vi "imagesurfacetest.vi"(10 "ROilevel":T1, 11 "ImageSrc":T2) -> (3 "ImageDst":T2(plugin-control))   [LabVIEW 2015]
uses:
  <vilib>/vision/Image Controls.llb/IMAQ Image.ctl
  ImageSurface.dll
  <vilib>/vision/NI_Vision_Development_Module.lvlib
panel:
  in  "Radius":i32=20
  in  "valueMin":i16
  in  "valueMax":i16=10000
  in  "SkipInvalidValue":bool=TRUE
  out "Return":i32
  out "Alpha 2":dbl=0.09707686755683868
  out "Beta 2":dbl=-0.07680741008059666
  out "Gamma 2":dbl=1309.996631781547
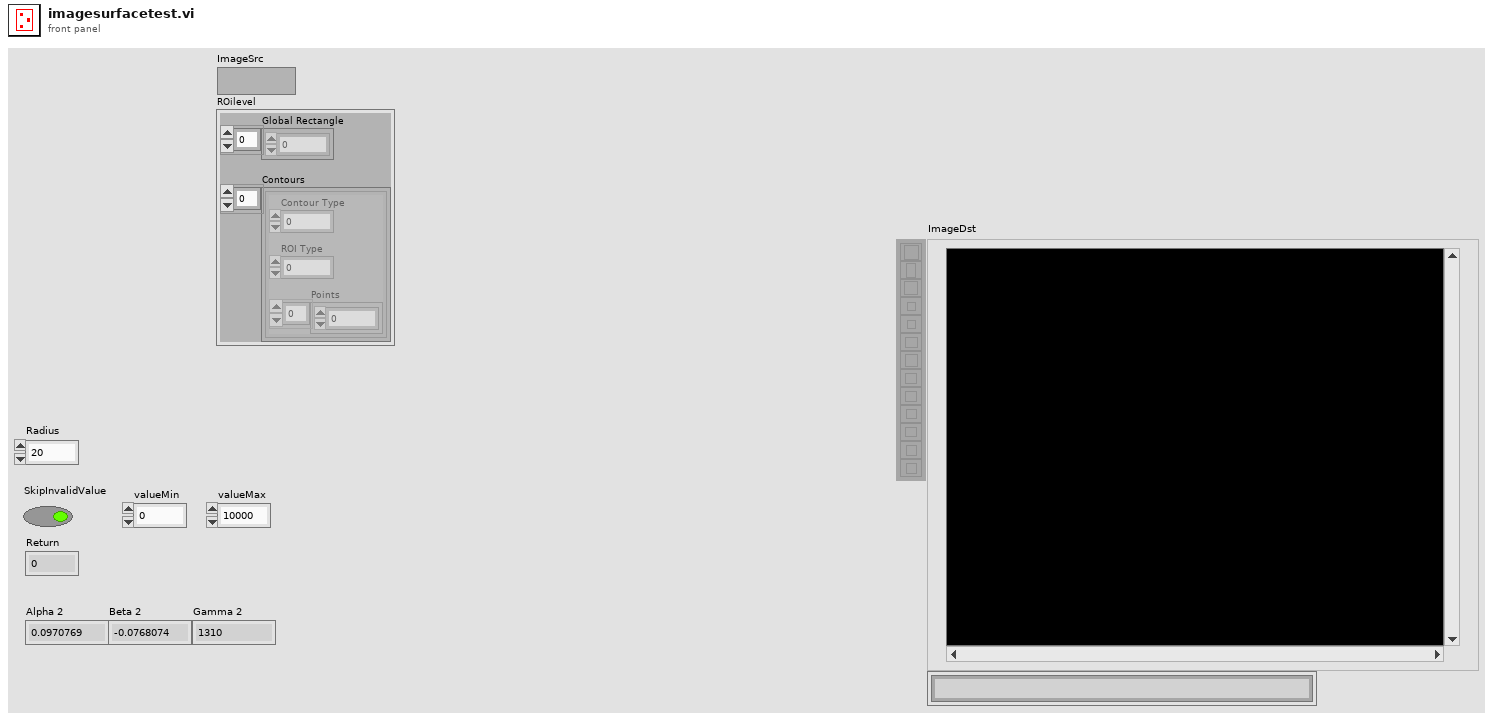
[diagram p1: front panel]
types:
  T1 = cluster{"Global Rectangle":i32[], "Contours":cluster{"Contour Type":u32, "ROI Type":u32, "Points":i32[]}[]}
  T2 = typedef "IMAQ Image.ctl" = refnum<image>
  T3 = cluster{"Contour Type":u32, "ROI Type":u32, "Points":i32[]}[]
  T4 = cluster{"Contour Type":u32, "ROI Type":u32, "Points":i32[]}
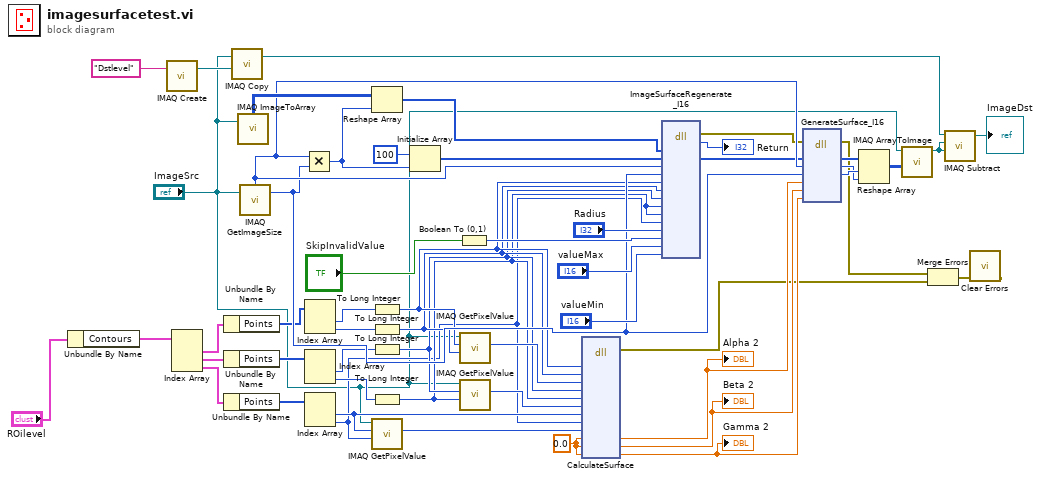
[diagram p0: block diagram]
diagram:
  w24 = 0.0 ("Gamma")
  n1 = Unbundle By Name("ROilevel") -> ("Contours"=w22:T3)
  n2 = call "IMAQ Create"("Image Name"="Dstlevel") -> ("New Image"=w7:T2)  [unwired: 4 in, 1 out]
  n3 = Index Array(array=w22) -> (element #1=w21:T4, element #2=w15:T4, element #3=w14:T4)  [unwired: 3 in]
  n4 = Unbundle By Name(w21) -> ("Points"=w20:i32[])
  n5 = Unbundle By Name(w15) -> ("Points"=w17:i32[])
  n6 = Unbundle By Name(w14) -> ("Points"=w16:i32[])
  n7 = call "IMAQ Copy"("Image Dst"=w7, "Image Src"="ImageSrc") -> ("Image Dst Out"=w5:T2)  [unwired: 4 in, 1 out]
  n8 = call "IMAQ ImageToArray"("Image"="ImageSrc") -> ("Image Pixels (U8)"=w53:u8[][])  [unwired: 3 in, 4 out]
  n9 = call "IMAQ GetImageSize"("Image"="ImageSrc") -> ("Y Resolution"=w35:i32, "X Resolution"=w36:i32)  [unwired: 3 in, 1 out]
  n10 = Multiply(x=w36, y=w35) -> (x*y=w45:i32)
  n11 = Index Array(array=w20) -> (element #1=w19:i32, element #2=w18:i32)  [unwired: 2 in]
  n12 = Index Array(array=w17) -> (element #1=w13:i32, element #2=w12:i32)  [unwired: 2 in]
  n13 = Index Array(array=w16) -> (element #1=w11:i32, element #2=w10:i32)  [unwired: 2 in]
  n14 = Reshape Array(w53, w45) -> (w48:u8[])
  n15 = To Long Integer(number=w19) -> (32bit integer=w28:i32)
  n16 = To Long Integer(number=w18) -> (32bit integer=w27:i32)
  n17 = To Long Integer(number=w13) -> (32bit integer=w26:i32)
  n18 = To Long Integer(number=w12) -> (32bit integer=w25:i32)
  n19 = call "IMAQ GetPixelValue"("Image"="ImageSrc", "X Coordinate"=w11, "Y Coordinate"=w10) -> ("Pixel Value (I16)"=w42:i16)  [unwired: 3 in, 4 out]
  n20 = Initialize Array(i16 100 ("元素"), w45) -> (w43:i16[])
  n21 = Boolean To (0,1)(Boolean="SkipInvalidValue") -> (0, 1=w51:i16)
  n22 = call "IMAQ GetPixelValue"("Image"="ImageSrc", "X Coordinate"=w28, "Y Coordinate"=w27) -> ("Pixel Value (I16)"=w40:i16)  [unwired: 3 in, 4 out]
  n23 = call "IMAQ GetPixelValue"("Image"="ImageSrc", "X Coordinate"=w26, "Y Coordinate"=w25) -> ("Pixel Value (I16)"=w41:i16)  [unwired: 3 in, 4 out]
  n24 = dll-call lib="PTH2^abs FAxxonSoftware WNC 20210822激光测量线激光3点校正平面ImageSurface.dll" fn="CalculateSurface"("X1"=w28, "Y1"=w27, "Z1"=w40, "X2"=w26, "Y2"=w25, "Z2"=w41, "X3"=w11, "Y3"=w10, "Z3"=w42, "Alpha"=w24, "Beta"=w24, "Gamma"=w24) -> (error out=w3:errorcluster, "Alpha"=w39:dbl, "Beta"=w38:dbl, "Gamma"=w37:dbl)  [unwired: 13 in, 1 out]
  "Alpha 2" <- w39
  "Beta 2" <- w38
  "Gamma 2" <- w37
  n25 = dll-call lib="PTH2^abs FAxxonSoftware WNC 20210822激光测量线激光3点校正平面ImageSurface.dll" fn="ImageSurfaceRegenerate_I16"("imageSrc"=w48, "imageDst"=w43, "nWidth"=w36, "nHeight"=w35, "nPoint1_X"=w28, "nPoint1_Y"=w27, "nPoint2_X"=w26, "nPoint2_Y"=w25, "nPoint3_X"=w25, "nPoint3_Y"=w10, "nDiamondRadius"="Radius", "bSkipInvalidValue"=w51, "valueMax"="valueMax", "valueMin"="valueMin") -> (error out=w4:errorcluster, "Return"=→"Return":i32, "imageDst"=w34:i16[])  [unwired: 16 in, 1 out]
  n26 = dll-call lib="PTH2^abs FAxxonSoftware WNC 20210822激光测量线激光3点校正平面ImageSurface.dll" fn="GenerateSurface_I16"(error in=w4, "imageDst"=w34, "nWidth"=w36, "nHeight"=w35, "Alpha"=w39, "Beta"=w38, "Gamma"=w37) -> (error out=w2:errorcluster, "imageDst"=w32:i16[], "nWidth"=w30:i32, "nHeight"=w31:i32)  [unwired: 6 in, 1 out]
  n27 = Reshape Array(w32, w31, w30) -> (w33:i16[][])
  n28 = call "IMAQ ArrayToImage"("Image Pixels (I16)"=w33, "Image"="ImageSrc") -> ("Image Out"=w29:T2)  [unwired: 8 in, 1 out]
  n29 = Merge Errors(w2, w3) -> (w1:errorcluster)
  n30 = call "IMAQ Subtract"("Image Src A"=w5, "Image Dst"=w29, "Image Src B"=w29) -> ("Image Dst Out"=→"ImageDst":T2)  [unwired: 4 in, 1 out]
  n31 = call <vilib>:"Clear Errors.vi"("error in (no error)"=w1) -> ()  [unwired: 5 in, 2 out]
